vi "get UI reference.vi"(8 "error in":errorcluster, 11 "VI modification in":refnum<class "VI modification.lvclass">=refnum) -> (0 "error out":errorcluster, 2 "VI Refnum":refnum<vi>, 3 "VI modification out":refnum<class "VI modification.lvclass">)   [LabVIEW 2013, in "VI modification.lvclass"]
uses:
  VI modification.lvclass
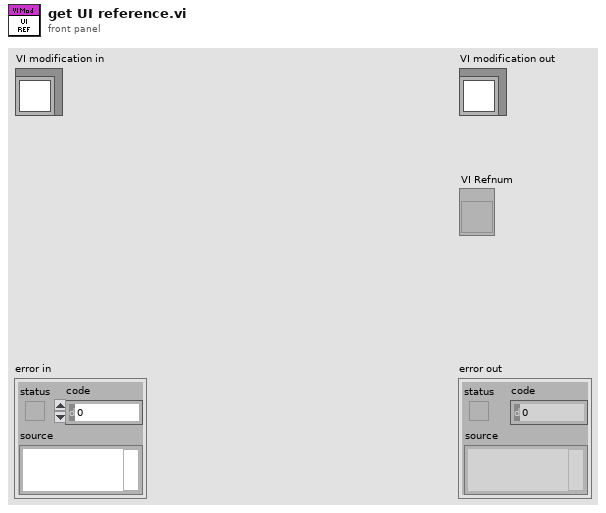
[diagram p1: front panel]
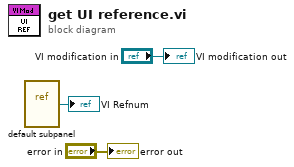
[diagram p0: block diagram]
diagram:
  n1 = vi-ref "default subpanel.vi"() -> (→"VI Refnum":refnum<vi>)
  "error out" <- "error in"
  "VI modification out" <- "VI modification in"
